vi "Global.vi"() -> ()   [LabVIEW 2010, in "CAN Log Transfer and Convert.lvlib"]
uses:
  CAN Log Transfer and Convert.lvlib
panel:
  out "Settings":refnum<vi>[](array[refnum])
  out "Abort Flag":bool
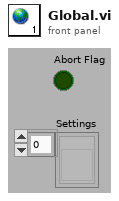
[diagram p1: front panel]
diagram:
